vi "ExportLog.vi"(4 "LogPath":path, 5 "Log Array":string[](array[string])) -> (0 "new file path (Not A Path if cancelled)":path, 2 "Log String":string)   [LabVIEW 2013]
uses:
  <vilib>/Utility/file.llb/Write To Spreadsheet File (string).vi
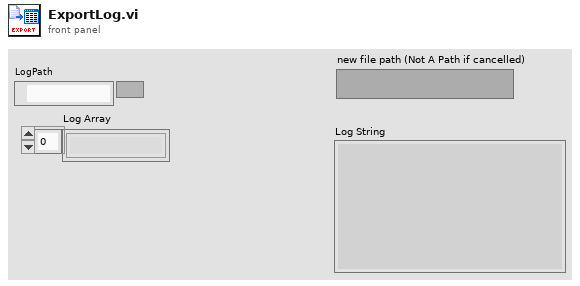
[diagram p1: front panel]
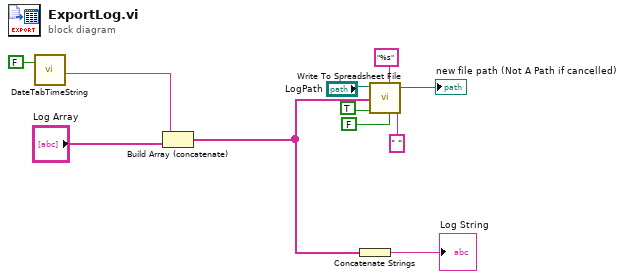
[diagram p0: block diagram]
diagram:
  n1 = call "DateTabTimeString.vi"("Seconds?"=FALSE) -> ("Date/Time String"=w10:string)  [unwired: 1 in]
  n2 = Build Array (concatenate)(w10, "Log Array") -> (w2:string[])
  n3 = Concatenate Strings(w2) -> (→"Log String":string)
  n4 = call-poly <vilib>:"Write To Spreadsheet File.vi"("delimiter (\\t)"=" " ("delimiter (\\t)"), "transpose? (no:F)"=FALSE, "format (%s)"="%s" ("format (%.3f)"), "append to file? (new file:F)"=TRUE, "1D data"=w2, "file path (dialog if empty)"="LogPath") -> ("new file path (Not A Path if cancelled)"=→"new file path (Not A Path if cancelled)":path)  [unwired: 2 in]
